vi "ReadAverageSpectrum.vi"(10 "Exposure (*2.375 ms)":u16=2, 11 "Average#":i32) -> (3 "Spectral Amplitude":dbl[](array[numeric]))   [LabVIEW 2022 SP3]
uses:
  <vilib>/Analysis/baseanly.llb/Mean (DBL).vi
  <vilib>/Analysis/NI_AALBase.lvlib
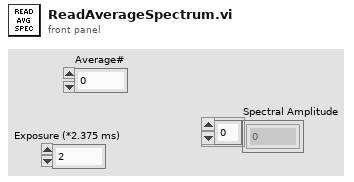
[diagram p1: front panel]
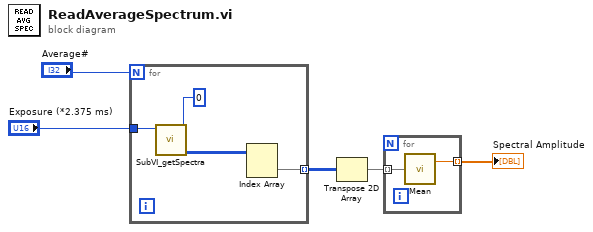
[diagram p0: block diagram]
diagram:
  n1 = for {
    N: "Average#" -> [_]
    tunnel: [w7] -> w3 mode=indexing
    tunnel: "Exposure (*2.375 ms)" -> [w6]
    n2 = call "SubVI_getSpectra.vi"("test1"=u8 0, "Exposure"=w6) -> ("all spectra"=w8:i16[][])  [unwired: 8 in, 1 out]
    n3 = Index Array(array=w8) -> (element=w7:i16[])  [unwired: 2 in]
  }
  n4 = Transpose 2D Array(2D array=w3) -> (transposed array=w2:i16[][])
  n5 = for {
    tunnel: [w10] -> w1 mode=indexing
    tunnel: w2 -> [w11] mode=indexing
    n6 = call-poly <vilib>:"Mean.vi"("X"=w11) -> ("mean"=w10:dbl)  [unwired: 1 out]
  }
  "Spectral Amplitude" <- w1
